vi "Write View Channel info.vi"(8 "error in":errorcluster, 10 "channel info":T1, 11 "channel in":refnum<class "_Channel.lvclass">) -> (0 "error out":errorcluster, 3 "channel out":refnum<class "_Channel.lvclass">)   [LabVIEW 2013, in "_Channel.lvclass"]
uses:
  _Channel.lvclass
  ChannelDisplayInfo.ctl
  _Channel.lvclass/_Channel.ctl
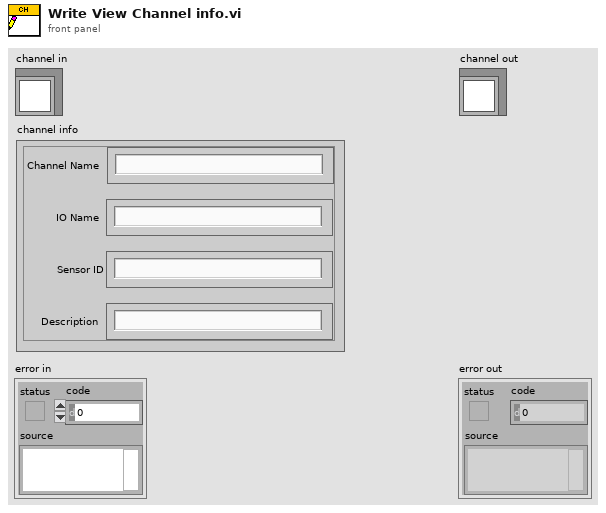
[diagram p1: front panel]
types:
  T1 = typedef "_Channel.lvclass/ChannelDisplayInfo.ctl" = cluster{"IO Name":string, "Sensor ID":string, "Channel Name":string, "Description ":string}
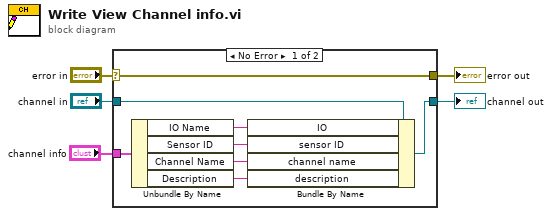
[diagram p0: block diagram]
diagram:
  n1 = case shown="No Error" "error in" {
    selector: "error in" -> [w13 w14]
    tunnel: [w13 w14] -> w4
    tunnel: [w7 w15] -> w2
    tunnel: "channel in" -> [w6 w15]
    tunnel: "channel info" -> [w8 _]
    frame No Error {
      n2 = Unbundle By Name(w8) -> ("IO Name"=w12:string, "Sensor ID"=w11:string, "Channel Name"=w10:string, "Description"=w9:string)
      n3 = Bundle By Name(cluster=w6, "IO"=w12, "sensor ID"=w11, "channel name"=w10, "description"=w9) -> (w7:refnum<class "_Channel.lvclass">)
    }
    frame Error {
    }
  }
  "error out" <- w4
  "channel out" <- w2
